vi "visionTarget.vi"(3 "Error In":errorcluster, 5 "Stop Button":bool) -> (0 "Error Out":errorcluster, 1 "it2(nut)":string, 2 "it1(screw)":string)   [LabVIEW 2019]
uses:
  WSCbot_V3_Toolkit.lvlibp
panel:
  out "finish?":bool
  out "Output":T1(plugin-control)
  out "Original":T1(plugin-control)
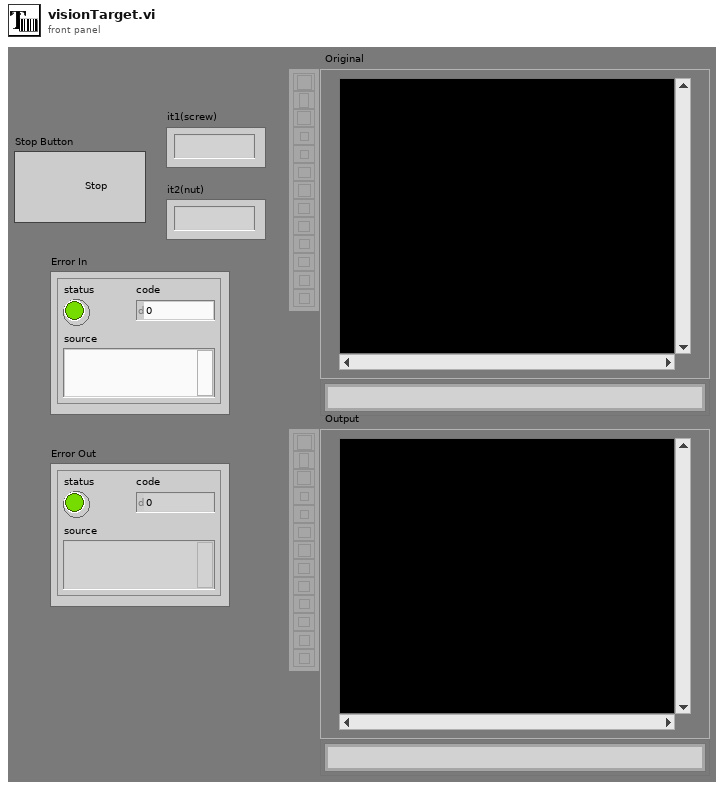
[diagram p1: front panel]
types:
  T1 = typedef "IMAQ Image.ctl" = refnum<image>
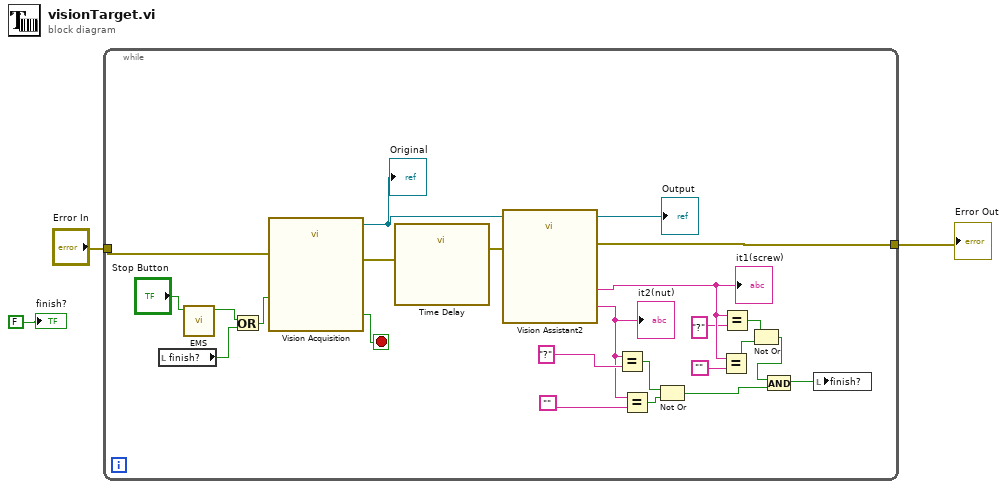
[diagram p0: block diagram]
diagram:
  n1 = while {
    tunnel: "Error In" -> [w8]
    tunnel: [w26] -> w2
    stop <- w6 stop-if-true
    n2 = local read "finish?"() -> (w9:bool)
    n3 = call "EMS.vi"("ProgramStop"="Stop Button") -> ("EMS"=w10:bool)  [unwired: 9 in, 1 out]
    n4 = Or(x=w10, y=w9) -> (x .or. y?=w5:bool)
    n5 = call "Vision Acquisition"("Stop (F)"=w5, "error in"=w8) -> ("Image Out"=w4:T1, "Stopped"=w6:bool, "error out"=w7:errorcluster)  [unwired: 23 in]
    "Original" <- w4
    n6 = call "Time Delay"("error in (no error)"=w7) -> ("error out"=w13:errorcluster)  [unwired: 10 in]
    n7 = call "Vision Assistant2"("Image In"=w4, "error in"=w13) -> ("Image Out"=→"Output":T1, "String (OCR/OCV 1)"=w20:string, "String (OCR/OCV 2)"=w24:string, "error out"=w26:errorcluster)  [unwired: 22 in]
    "it1(screw)" <- w20
    "it2(nut)" <- w24
    n8 = Equal?(x=w24, y="?") -> (x = y?=w22:bool)
    n9 = Equal?(x=w24, y="") -> (x = y?=w21:bool)
    n10 = Not Or(1:w21, 2:w22) -> (0:w15:bool)
    n11 = Equal?(x=w20, y="") -> (x = y?=w16:bool)
    n12 = Equal?(x=w20, y="?") -> (x = y?=w17:bool)
    n13 = Not Or(1:w16, 2:w17) -> (0:w14:bool)
    n14 = And(x=w14, y=w15) -> (x .and. y?=w11:bool)
    n15 = local write "finish?"(w11) -> ()
  }
  "Error Out" <- w2
  "finish?" <- FALSE ("Boolean")
